vi "Send Command.vi"(8 "error in":errorcluster, 9 "Value":variant, 10 "Command":string, 11 "PRM in":refnum<class "PRM.lvclass">) -> (0 "error out":errorcluster, 3 "PRM out":refnum<class "PRM.lvclass">)   [LabVIEW 2019, in "PRM.lvlib" / "PRM.lvclass"]
uses:
  Library/PRM.lvclass
  C:/Users/Public/Documents/Development/builds/Engine/Engine.lvlibp/Project/Engine.lvclass
  C:/Users/Public/Documents/Development/builds/Engine/Monitored Actor.lvlibp/Monitored Actor/Monitored Actor/Monitored Actor.lvclass
  builds/Engine/Engine.lvlibp/Accessors/Read Self Q.vi
  builds/Engine/Monitored Actor.lvlibp/Monitored Actor/Monitored Actor/Read Actor Label.vi
  <vilib>/Utility/error.llb/Error Cluster From Error Code.vi
  builds/Engine/Actor Framework.lvlibp/1abvi3w/vi.lib/ActorFramework/Message Enqueuer/Message Enqueuer.lvclass
  <vilib>/ErrorRing/Error Ring.xnode
  builds/Engine/Engine.lvlibp/Project/Engine.lvclass
  PRM Messages/Set Channel by Name Msg/Set Channel by Name Msg.lvclass
  C:/Users/Public/Documents/Development/builds/Instruments/Instruments.lvlibp/Library/Instruments.lvclass
  C:/Users/Public/Documents/Development/builds/Tools/Config.lvlibp/Config.lvclass
  C:/Users/Public/Documents/Development/builds/Engine/State Actor.lvlibp/Library/State Actor.lvclass
  C:/Users/Public/Documents/Development/builds/Engine/Panel Manager.lvlibp/Panel Actor/Panel Actor.lvclass
  C:/Users/Public/Documents/Development/builds/Engine/Actor Framework.lvlibp/1abvi3w/vi.lib/ActorFramework/Actor/Actor.lvclass
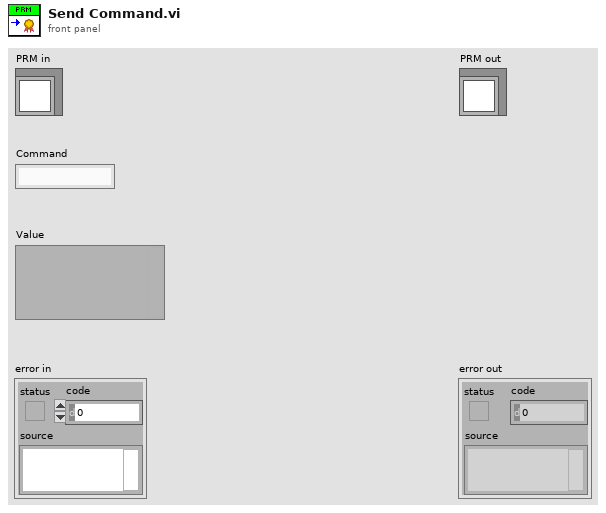
[diagram p1: front panel]
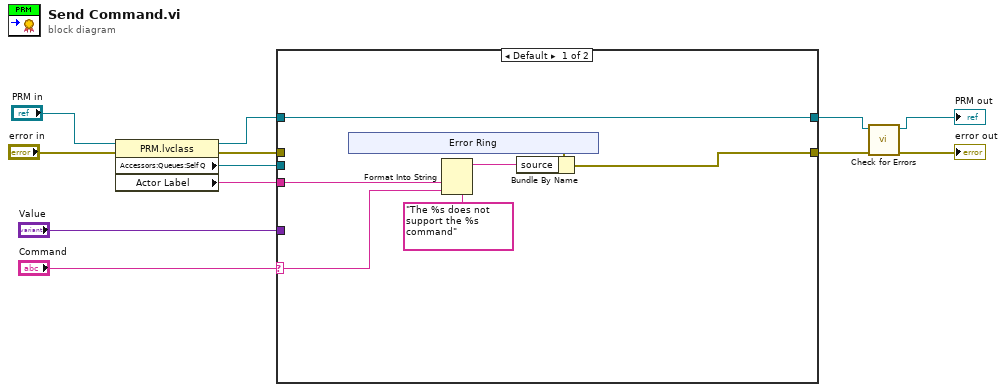
[diagram p0: block diagram]
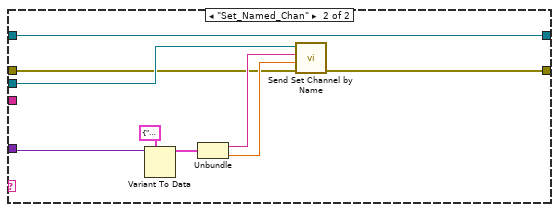
[diagram p2: hidden frame]
diagram:
  n1 = property class="PRM.lvclass"(reference="PRM in", error in="error in") -> (reference out=w8:refnum<class "PRM.lvclass">, error out=w5:errorcluster, "Accessors:Queues:Self Q"=w9:refnum<class "Message Enqueuer.lvclass">, "Actor Label"=w7:string)
  n2 = case shown="Default" "Command" {
    selector: "Command" -> [w16 _]
    tunnel: "Value" -> [_ w30]
    tunnel: w9 -> [_ w31]
    tunnel: [w13 w32] -> w2
    tunnel: w8 -> [w13 w32]
    tunnel: w7 -> [w15 _]
    tunnel: [w14 w24] -> w4
    tunnel: w5 -> [_ w25]
    frame Default {
      n3 = xnode "Error Ring"() -> ("error out"=w17:errorcluster)
      n4 = Format Into String(format string="The %s does not support the %s command", w15, w16) -> (resulting string=w18:string)  [unwired: 2 in, 1 out]
      n5 = Bundle By Name(cluster=w17, "source"=w18) -> (w14:errorcluster)
    }
    frame "Set_Named_Chan" {
      n6 = Variant To Data(type=cluster{"Name":string, "Target":dbl} {"Name"="", "Target"=0.0}, Variant=w30) -> (data=w28:cluster{"Name":string, "Target":dbl})  [unwired: 1 in, 1 out]
      n7 = Unbundle(w28) -> ("Name"=w27:string, "Target"=w26:dbl)
      n8 = call "Send Set Channel by Name.vi"("error in (no error)"=w25, "Target"=w26, "Channel Name"=w27, "Message Enqueuer"=w31) -> ("error out"=w24:errorcluster)  [unwired: 6 in, 1 out]
    }
  }
  n9 = call "Check for Errors.vi"("error in"=w4, "Engine in"=w2) -> ("error out"=→"error out":errorcluster, "Engine out"=→"PRM out":refnum<class "PRM.lvclass">)  [unwired: 8 in]
